vi "readDAQ.vi"(8 "error in (no error)":errorcluster, 11 "DAQ in":refnum<class "DAQ.lvclass">) -> (0 "error out":errorcluster, 2 "señal":waveform(dbl)[](array[waveform]), 3 "DAQ out":refnum<class "DAQ.lvclass">)   [LabVIEW 2019, in "DAQ.lvclass"]
uses:
  DAQ.lvclass
  DAQ.lvclass/DAQ.ctl
  <vilib>/DAQmx/read.llb/DAQmx Read (Analog 1D Wfm NChan NSamp).vi
  <vilib>/DAQmx/miscellaneous.llb/DAQmx Fill In Error Info.vi
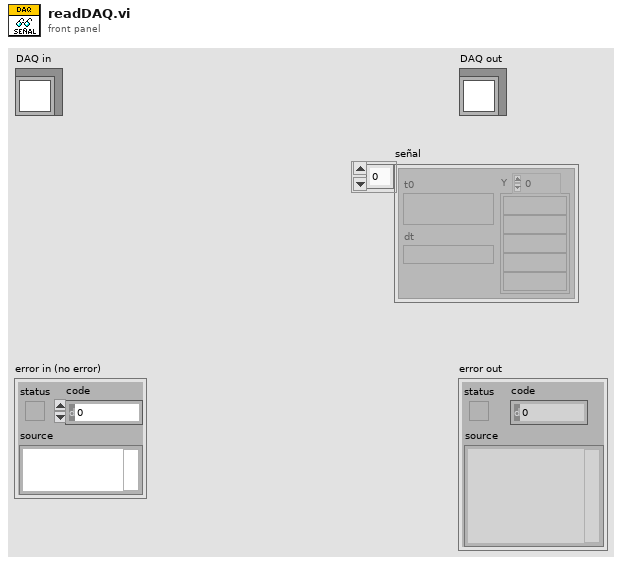
[diagram p1: front panel]
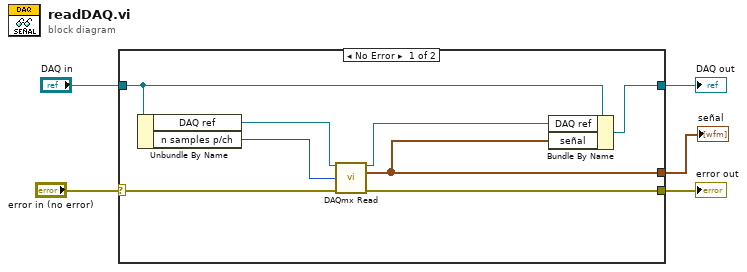
[diagram p0: block diagram]
diagram:
  n1 = case shown="No Error" "error in (no error)" {
    selector: "error in (no error)" -> [w12 w15]
    tunnel: [w8 w15] -> w4
    tunnel: [w9 w14] -> w2
    tunnel: "DAQ in" -> [w10 w14]
    tunnel: [w6 _] -> w1
    frame No Error {
      n2 = Unbundle By Name(w10) -> ("DAQ ref"=w13:refnum<k21>, "n samples p/ch"=w7:i32)
      n3 = call-poly <vilib>:"DAQmx Read.vi"("task/channels in"=w13, "number of samples per channel"=w7, "error in"=w12) -> ("task out"=w11:refnum<k21>, "data"=w6:waveform(dbl)[], "error out"=w8:errorcluster)  [unwired: 10 in]
      n4 = Bundle By Name(cluster=w10, "DAQ ref"=w11, "señal"=w6) -> (w9:refnum<class "DAQ.lvclass">)
    }
    frame Error {
    }
  }
  "error out" <- w4
  "DAQ out" <- w2
  "señal" <- w1
